vi "Ch Set FPDIV.vi"(7 "DIV":u16, 9 "FP":u16, 10 "Channel":u8, 11 "devId":i32) -> (2 "devId out":i32, 3 "function return":i32)   [LabVIEW 2013, in "CHR34XXX.lvlib"]
doc: "DLL BOOL __stdcall CHR34XXX_Ch_SetCommState(IN int devId,IN BYTE Channel,IN pCHRUART_DCB_ST pstRsdcb); DLL BOOL __stdcall CHR34XXX_Ch_SetFPDIV(IN int devId,IN BYTE Channel,IN WORD FP,IN WORD DIV);"
uses:
  CHR34XXX.lvlib
  CHR34XXX.dll
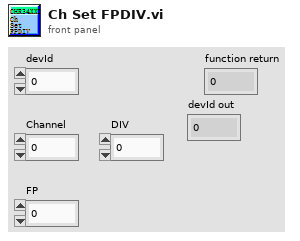
[diagram p1: front panel]
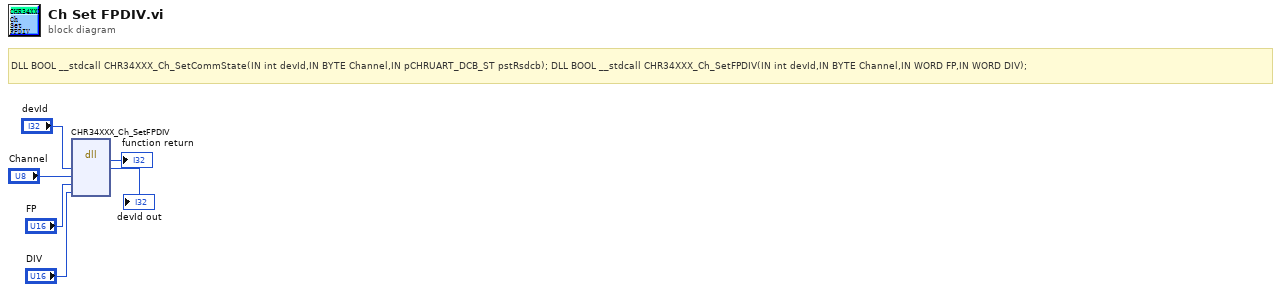
[diagram p0: block diagram]
diagram:
  # "DLL BOOL __stdcall CHR34XXX_Ch_SetCommState(IN int devId,IN BYTE Channel,IN pCHRUART_DCB_ST pstRsdcb); DLL BOOL __stdcall CHR34XXX_Ch_SetFPDIV(IN int devId,IN BYTE Channel,IN WORD FP,IN WORD DIV);"
  n1 = dll-call lib="C:/Users/Administrator/Desktop/CHR34XXX_lv/lv_lib/CHR34XXX.*" fn="CHR34XXX_Ch_SetFPDIV"("devId"="devId", "Channel"="Channel", "FP"="FP", "DIV"="DIV") -> (→"function return":i32, "devId"=→"devId out":i32)  [unwired: 6 in, 2 out]
